vi "ClsGetLastSampleMultiChannelDevice.vi"(8 "error in":errorcluster, 11 "Connection In":u32) -> (0 "error out":errorcluster, 1 "Peak Signals":dbl[][](array[numeric]), 2 "Global Signals":dbl[](array[numeric]), 3 "Connection Out":u32, 5 "Have data?":bool)   [LabVIEW 2015]
doc: "Get Last Sample Multi Channel:\n\nThis function is used for MPS/CLS devices. This function is used to get the last/newest valid sample from device(which may be duplicated for several consecutive calls if no newer sample is available). By calling this function, client will also jump to the last valid position in the data buffer used to temporarily store the data from device. Note that this function is none-block which means it will return immediately no matter if there is any data available.\n\nConnection In[Input]: the connection handle which is initially created by Open Connection subVI.\n\nHave data?[Output]: since this subVI is none-block which will return immediately with an empty data array if there is no data available, this boolean output is used for indicating whether there is any data in the output at all.\n\nGlobal Signals[Output]: The one dimensional array for global signals data. Global signals are those who occurs only once for all the channels per sample. Examples of global signals include sample counter, StartTime, EncX Start Pos and EncY Start Pos, etc.. Note that you can use Get Output Signal IDs subVI to see the ordering of signal IDs correspondent to this data array. For example, if the Get Output Signal IDs subVI returns the signal IDs are 83 85 16640 16642, then the global signals array here are ordered as signal IDs 83 85. If there is no data, an empty array will be returned.\n\nPeak Signals[Output]: The two dimensional array for peak signals data. Peak signals are those who occur only once for each channel per sample. Peak signals include Peak Position, Quality, CCD Satuation, CCD Position, Median and Peak Width. For the 2D data array, dimension 1 is for channels and dimension 2 is for different peak signals. Note that you can use Get Signal IDs subVI to see the ordering of peak signal IDs correspondent to this data array. For example, if the Get Output Signal IDs subVI returns the signal IDs are 83 85 16640 16642, then the signals order (second dimension) of peak signals array here are ordered as signal IDs 16640 16642. If there is no data, an empty array will be returned.\n\nConnection Out[Output]: the connection handle output which could be used for next subVI refering to the same connection."
uses:
  dependent dlls/CHRocodileDLL.dll
panel:
  out "Number of Peak signals per Channel":dbl
  out "_pnNumberOfSignals":i32
  out "_pnNumberOfGlobalSigs":i32
  out "_pnNumberOfChannels":i32
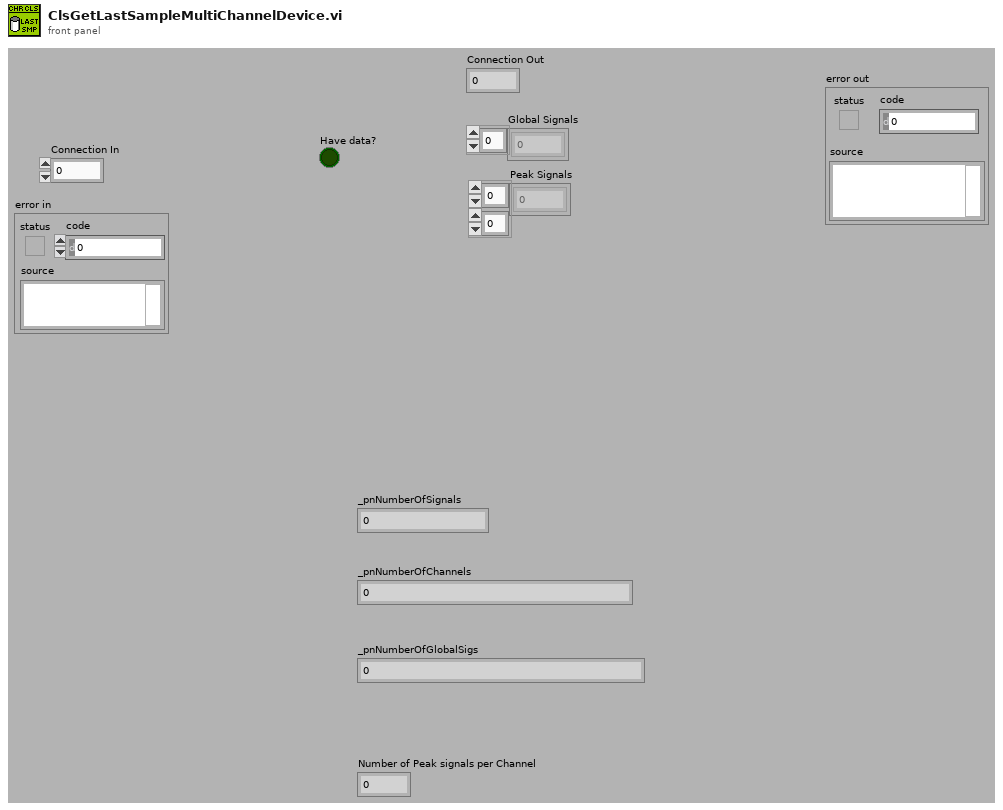
[diagram p1: front panel]
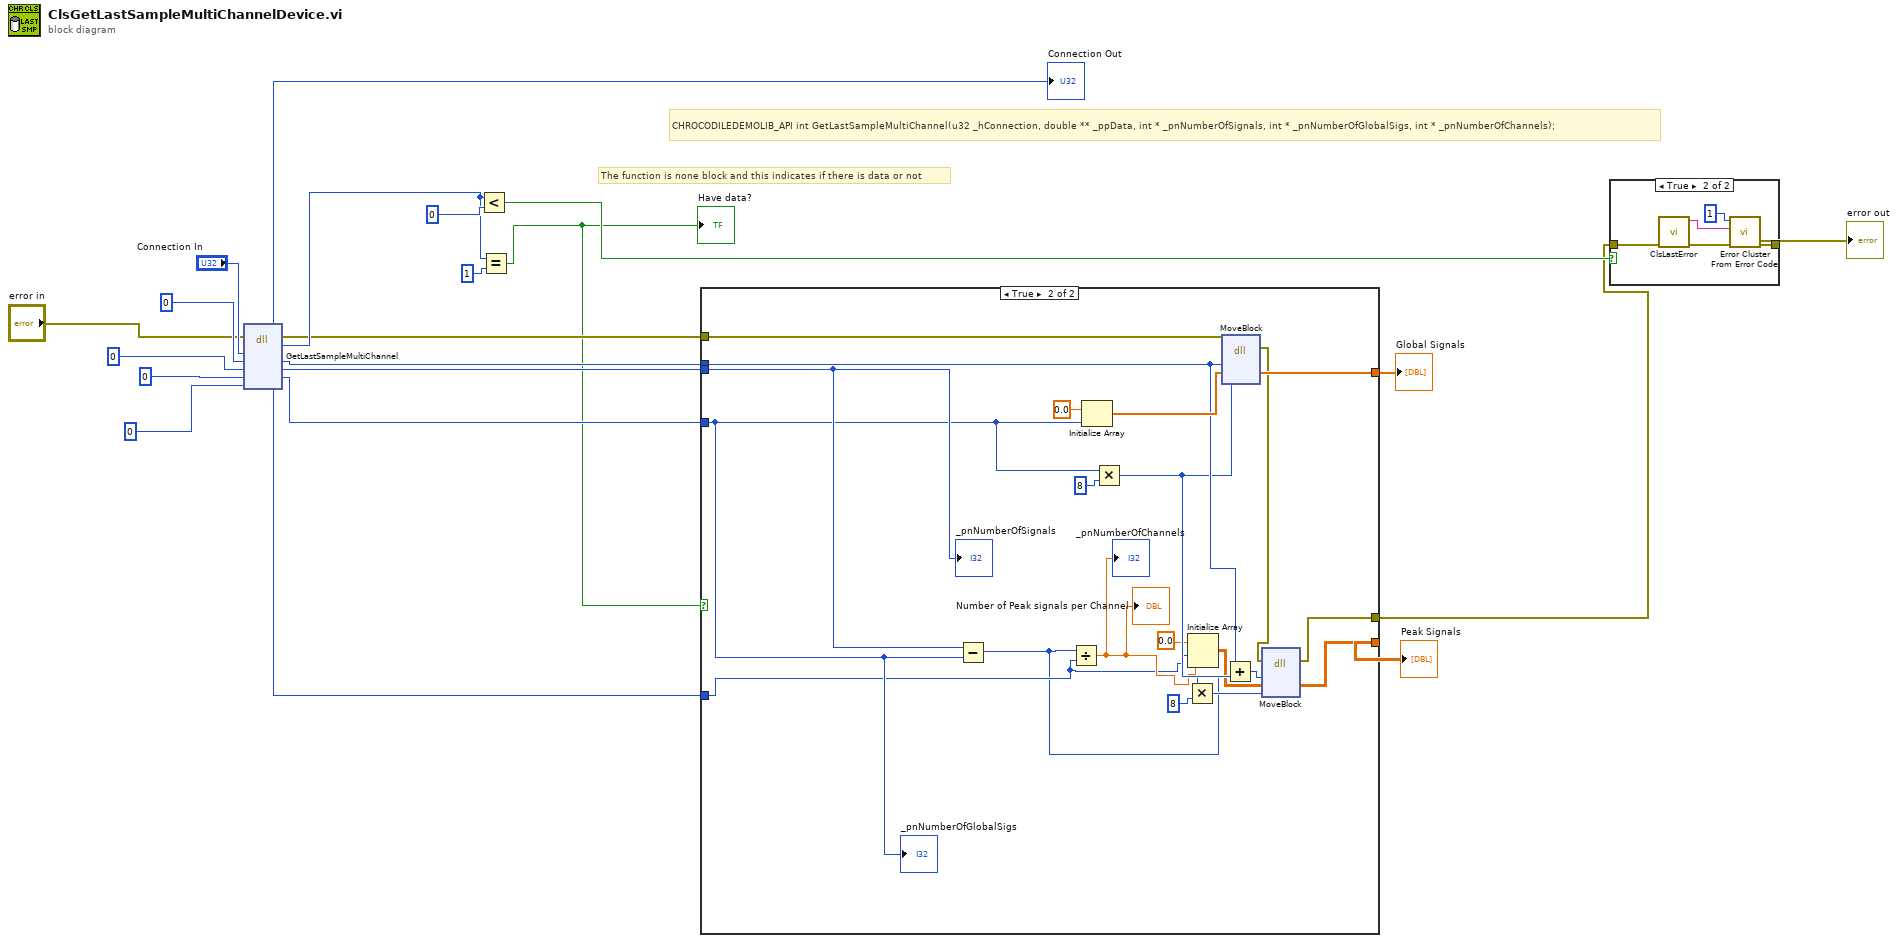
[diagram p0: block diagram]
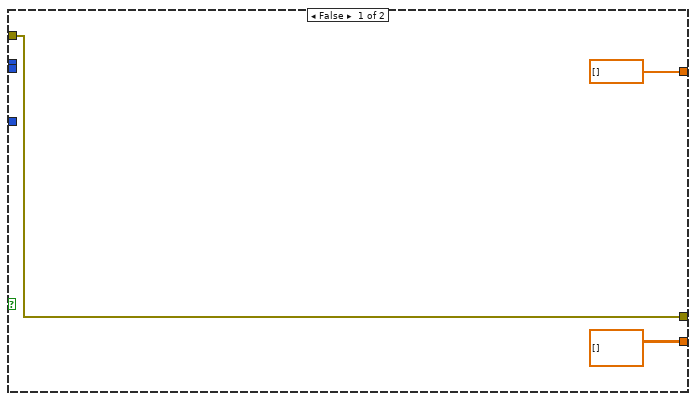
[diagram p2: hidden frame]
diagram:
  # "The function is none block and this indicates if there is data or not"
  # "CHROCODILEDEMOLIB_API int GetLastSampleMultiChannel(u32 _hConnection, double ** _ppData, int * _pnNumberOfSignals, int * _pnNumberOfGlobalSigs, int * _pnNumberOfChannels);"
  n1 = dll-call lib="C:/Users/privat/Documents/ADP-SLA/Drop Impact Teststand/dependent dlls/CHRocodileDLL.dll" fn="GetLastSampleMultiChannel"(error in="error in", "_hConnection"="Connection In", "_ppData"=i64 0, "_pnNumberOfSignals"=0, "_pnNumberOfGlobalSigs"=0, "_pnNumberOfChannels"=0) -> (error out=w5:errorcluster, "return type"=w8:i32, "_hConnection"=→"Connection Out":u32, "_ppData"=w14:i64, "_pnNumberOfSignals"=w13:i32, "_pnNumberOfGlobalSigs"=w12:i32, "_pnNumberOfChannels"=w2:i32)  [unwired: 2 in, 1 out]
  n2 = Less?(x=w8, y=0) -> (x < y?=w6:bool)
  n3 = Equal?(x=w8, y=1) -> (x = y?=w1:bool)
  "Have data?" <- w1
  n4 = case shown="True" w1 {
    tunnel: [dbl[] [] ("Destination") w41] -> w16
    tunnel: [dbl[][] [] ("Destination") w40] -> w15
    tunnel: w14 -> [_ w39]
    tunnel: w13 -> [_ w36]
    tunnel: w12 -> [_ w35]
    tunnel: w5 -> [w22 w30]
    tunnel: [w22 w28] -> w4
    tunnel: w2 -> [_ w26]
    frame False {
    }
    frame True {
      n5 = Subtract(x=w36, y=w35) -> (x-y=w25:i32)
      n6 = Divide(x=w25, y=w26) -> (x/y=w27:dbl)
      "_pnNumberOfChannels" <- w27
      "Number of Peak signals per Channel" <- w27
      n7 = Initialize Array(0.0 ("element"), w35) -> (w42:dbl[])
      n8 = Multiply(x=w35, y=8) -> (x*y=w38:i32)
      n9 = Multiply(x=w25, y=8) -> (x*y=w31:i32)
      n10 = Initialize Array(0.0 ("element"), w26, w27) -> (w33:dbl[][])
      n11 = dll-call lib="LabVIEW" fn="MoveBlock"(error in=w30, "Address(pointer)"=w39, "Destination"=w42, "Size"=w38) -> (error out=w29:errorcluster, "Destination"=w41:dbl[])  [unwired: 5 in, 1 out]
      n12 = Add(x=w39, y=w38) -> (x+y=w37:i64)
      n13 = dll-call lib="LabVIEW" fn="MoveBlock"(error in=w29, "Address(pointer)"=w37, "Destination"=w33, "Size"=w31) -> (error out=w28:errorcluster, "Destination"=w40:dbl[][])  [unwired: 5 in, 1 out]
      "_pnNumberOfGlobalSigs" <- w35
      "_pnNumberOfSignals" <- w36
    }
  }
  "Global Signals" <- w16
  "Peak Signals" <- w15
  n14 = case shown="True" w6 {
    tunnel: [w45 w49] -> w7
    tunnel: w4 -> [w45 w46]
    frame False {
    }
    frame True {
      n15 = call "ClsLastError.vi"("error in (no error)"=w46) -> ("error out"=w47:errorcluster, "Error Message"=w48:string)  [unwired: 9 in]
      n16 = call <vilib>:"Error Cluster From Error Code.vi"("error in (no error)"=w47, "error message (\"\")"=w48, "error code (0)"=1) -> ("error out"=w49:errorcluster)  [unwired: 6 in]
    }
  }
  "error out" <- w7
